vi "RetrieveAcPwrMeasurementData.vi"(0 "WaveformChartReference":refnum<vi>, 1 "PlotYScale":u32[](array[numeric]), 5 "WaveformArrayIn":waveform(dbl)[](array[waveform]), 11 "error in (no error)":errorcluster) -> (4 "WaveformArrayOut":waveform(dbl)[](array[waveform]), 6 "OutputString(Chroma)":string, 8 "Incorrect DataType?":bool, 10 "Status Byte Register(NHRRGS)":T1(array[cluster]), 15 "error out":errorcluster)   [LabVIEW 2018, in "AcPwrShared.lvlib"]
doc: "This VI takes in the measurement data from an AcPwr Plugin and retrieves additional information from the attributes defined in the AcPwrAttriutesTypeDef.ctl such as Register Status Byte."
uses:
  AcPwrShared.lvlib
  clAcPwrAttributes.ctl
panel:
  out "Processing Time":u32
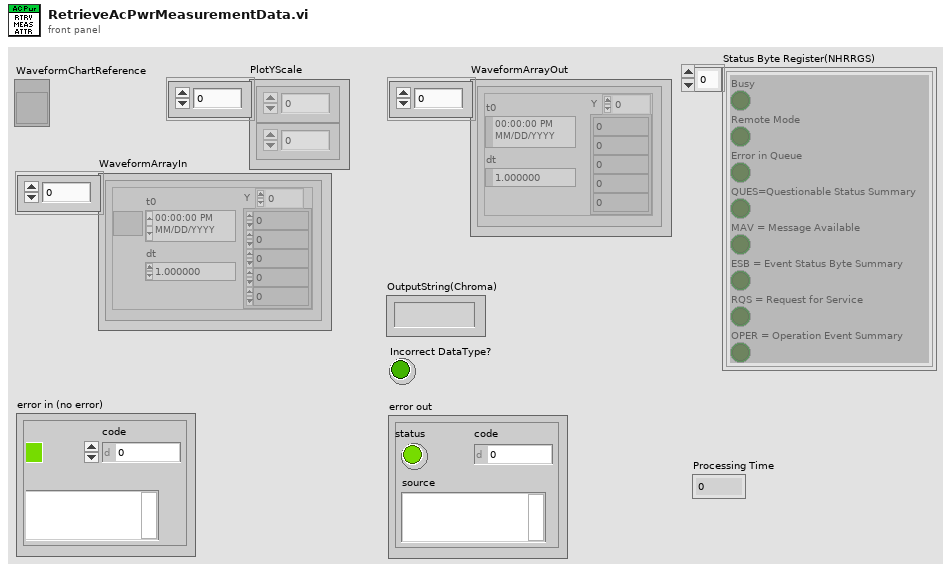
[diagram p1: front panel]
types:
  T1 = cluster{"Busy":bool, "Remote Mode":bool, "Error in Queue":bool, "QUES=Questionable Status Summary":bool, "MAV = Message Available":bool, "ESB = Event Status Byte Summary":bool, "RQS = Request for Service":bool, "OPER = Operation Event Summary":bool}[]
  T2 = typedef "AcPwrShared.lvlib/clAcPwrAttributes.ctl" = cluster{"ProtectionStatusString":string, "Handle_MeasurementType":string, "Status Byte Register":cluster{"Busy":bool, "Remote Mode":bool, "Error in Queue":bool, "QUES=Questionable Status Summary":bool, "MAV = Message Available":bool, "ESB = Event Status Byte Summary":bool, "RQS = Request for Service":bool, "OPER = Operation Event Summary":bool}}
  T3 = cluster{"Busy":bool, "Remote Mode":bool, "Error in Queue":bool, "QUES=Questionable Status Summary":bool, "MAV = Message Available":bool, "ESB = Event Status Byte Summary":bool, "RQS = Request for Service":bool, "OPER = Operation Event Summary":bool}
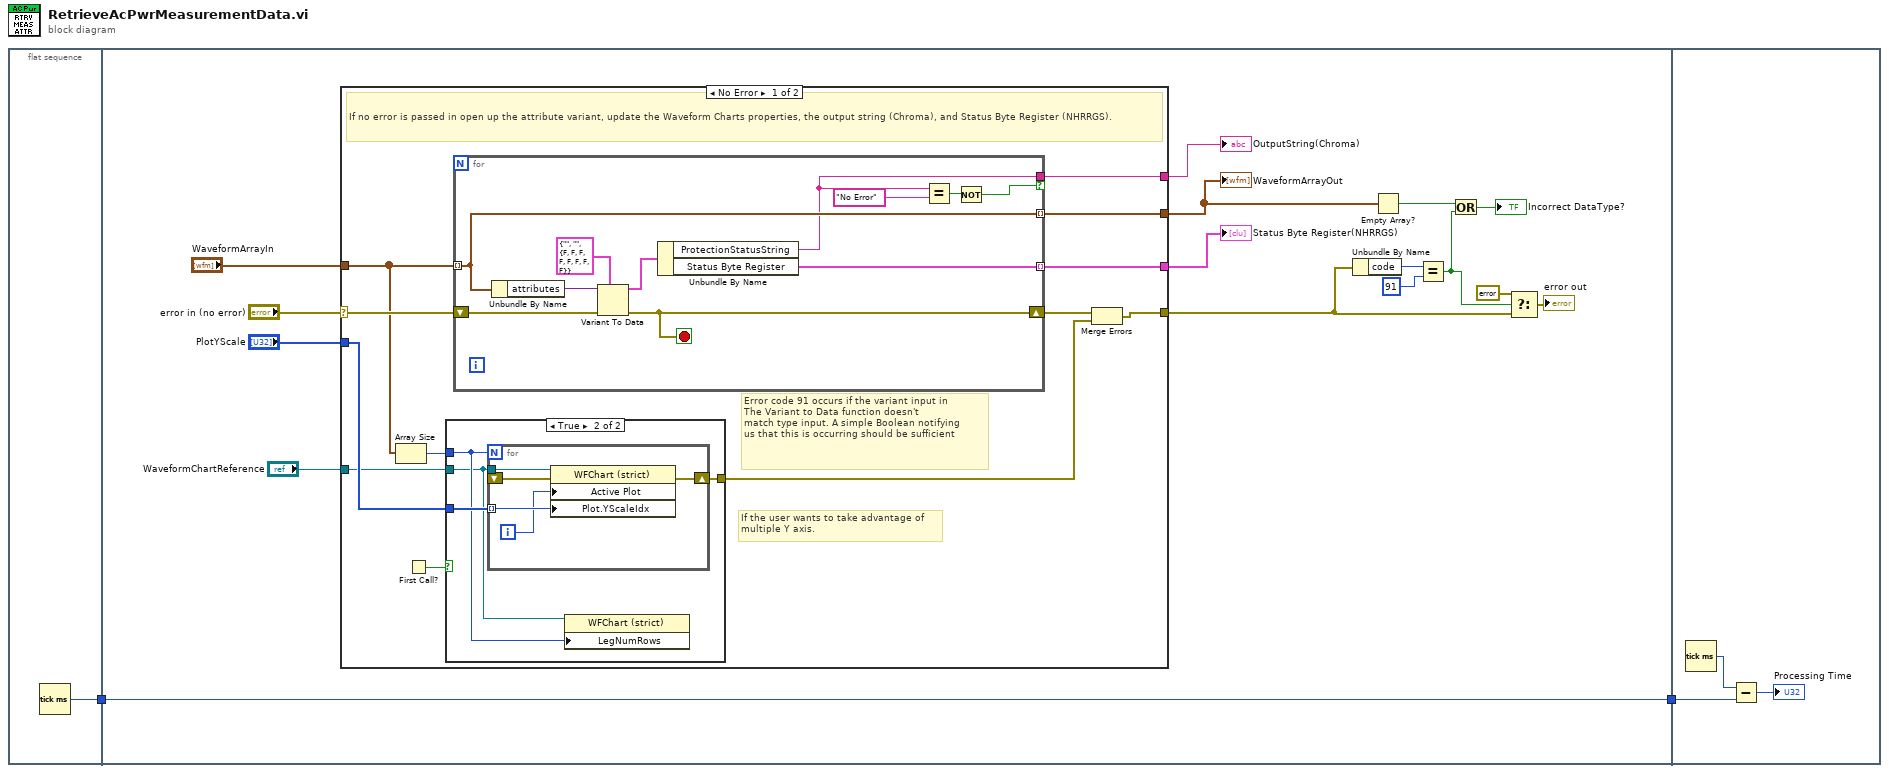
[diagram p0: block diagram]
diagram:
  n1 = flat-sequence {
    tunnel: [w3] -> w2
    tunnel: w2 -> [w4]
    tunnel: [w4] -> w1
    tunnel: w1 -> [w54]
    frame #0 {
      n2 = Tick Count (ms)() -> (millisecond timer value=w3:u32)
    }
    frame #1 {
      n3 = case shown="No Error" "error in (no error)" {
        selector: "error in (no error)" -> [w31 w52]
        tunnel: [w26 w52] -> w11
        tunnel: [w29 _] -> w8
        tunnel: "WaveformChartReference" -> [w23 _]
        tunnel: "PlotYScale" -> [w24 _]
        tunnel: [w28 _] -> w16
        tunnel: "WaveformArrayIn" -> [w21 _]
        tunnel: [w27 _] -> w9
        frame No Error {
          # "If the user wants to take advantage of \nmultiple Y axis."
          # "Error code 91 occurs if the variant input in \nThe Variant to Data function doesn't \nmatch type input. A simple Boolean notifying \nus that this is occurring should be sufficient"
          # "If no error is passed in open up the attribute variant, update the Waveform Charts properties, the output string (Chroma), and Status Byte Register (NHRRGS)."
          n4 = Array Size(array=w21) -> (size(s)=w20:i32)
          n5 = First Call?() -> (First Call?: T/F=w22:bool)
          n6 = case shown="True" w22 {
            tunnel: [_ w35] -> w25
            tunnel: w24 -> [_ w34]
            tunnel: w23 -> [_ w32]
            tunnel: w20 -> [_ w33]
            frame False {
            }
            frame True {
              n7 = for {
                N: w33 -> [_]
                tunnel: w32 -> [w36]
                tunnel: w34 -> [w40] mode=indexing
                shift-right: [w39] -> w35
                shift-left: _ -> [w38]
                i -> [w37]
                n8 = property on="Property Node" class="WFChart (strict)"(reference=w36, error in=w38, "Active Plot"=w37, "Plot.YScaleIdx"=w40) -> (error out=w39:errorcluster)  [unwired: 1 out]
              }
              n9 = property on="Property Node" class="WFChart (strict)"(reference=w32, "LegNumRows"=w33) -> ()  [unwired: 1 in, 2 out]
            }
          }
          n10 = for {
            shift-right: [w41] -> w30
            shift-left: w31 -> [w47]
            tunnel: [w49] -> w29 mode=indexing
            tunnel: [w43] -> w28 if=w46
            tunnel: w21 -> [w49] mode=indexing
            tunnel: [w42] -> w27 mode=indexing
            stop <- w41 stop-if-true
            n11 = Unbundle By Name(w49) -> ("attributes"=w48:variant)
            n12 = Variant To Data(error in=w47, type=T2 {"ProtectionStatusString"="", "Handle_MeasurementType"="", "Status Byte Register"={"Busy"=FALSE, "Remote Mode"=FALSE, "Error in Queue"=FALSE, "QUES=Questionable Status Summary"=FALSE, "MAV = Message Available"=FALSE, "ESB = Event Status Byte Summary"=FALSE, "RQS = Request for Service"=FALSE, "OPER = Operation Event Summary"=FALSE}} ("Attributes"), Variant=w48) -> (data=w44:T2, error out=w41:errorcluster)
            n13 = Unbundle By Name(w44) -> ("ProtectionStatusString"=w43:string, "Status Byte Register"=w42:T3)
            n14 = Equal?(x=w43, y="No Error") -> (x = y?=w51:bool)
            n15 = Not(x=w51) -> (.not. x?=w46:bool)
          }
          n16 = Merge Errors(w30, w25) -> (w26:errorcluster)
        }
        frame Error {
        }
      }
      "OutputString(Chroma)" <- w16
      "WaveformArrayOut" <- w8
      "Status Byte Register(NHRRGS)" <- w9
      n17 = Unbundle By Name(w11) -> ("code"=w15:i32)
      n18 = Empty Array?(array=w8) -> (empty?=w7:bool)
      n19 = Equal?(x=w15, y=91) -> (x = y?=w6:bool)
      n20 = Or(x=w7, y=w6) -> (x .or. y?=→"Incorrect DataType?":bool)
      n21 = Select(t=errorcluster {"status"=FALSE, "code"=0, "source"=""} ("error IO"), s=w6, f=w11) -> (s? t:f=→"error out":errorcluster)
    }
    frame #2 {
      n22 = Tick Count (ms)() -> (millisecond timer value=w55:u32)
      n23 = Subtract(x=w55, y=w54) -> (x-y=→"Processing Time":u32)
    }
  }
